vi "Save Encoder Data From MyRio_sub_VI.vi"() -> (3 "Output String":string)   [LabVIEW 2017]
panel:
  # "Save Encoder Data From MyRio_sub_VI.vi instructions:\n1. Run VI after main code has finished running\n2. Select location to save file in file dialog. Add .csv ending to filename.\n3. Click save"
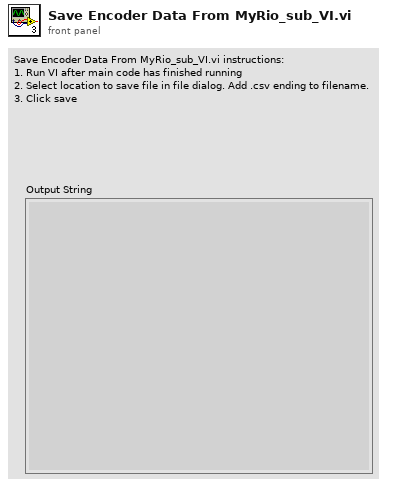
[diagram p1: front panel]
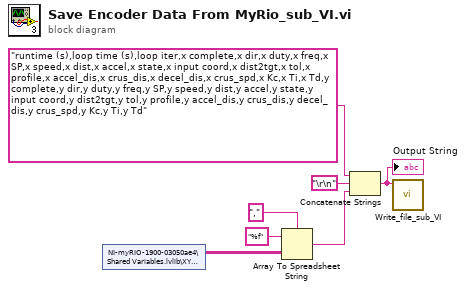
[diagram p0: block diagram]
diagram:
  n1 = shared-variable "NI-myRIO-1900-03050ae4\\Shared Variables.lvlib\\XY Datalog"() -> (w1:string[][])  [unwired: 1 in, 1 out]
  n2 = Array To Spreadsheet String(delimiter (Tab)=",", array=w1, 3:"%f" ("format string")) -> (spreadsheet string=w7:string)
  n3 = Concatenate Strings("runtime (s),loop time (s),loop iter,x complete,x dir,x duty,x freq,x SP,x speed,x dist,x accel,x state,x input coord,x dist2tgt,x tol,x profile,x accel_dis,x crus_dis,x decel_dis,x crus_spd,x Kc,x Ti,x Td,y complete,y dir,y duty,y freq,y SP,y speed,y dist,y accel,y state,y input coord,y dist2tgt,y tol,y profile,y accel_dis,y crus_dis,y decel_dis,y crus_spd,y Kc,y Ti,y Td", "\r\n", w7) -> (w6:string)
  "Output String" <- w6
  n4 = call "Write_file_sub_VI.vi"("Output String"=w6) -> ()  [unwired: 9 in, 2 out]
